vi "Script VeriStand Model core.vi"(9 "release/debug?":bool, 10 "build?":bool, 11 "VI path":path) -> (0 "error out":errorcluster)   [LabVIEW 2015, in "CD model script.lvlib"]
uses:
  CD model script.lvlib
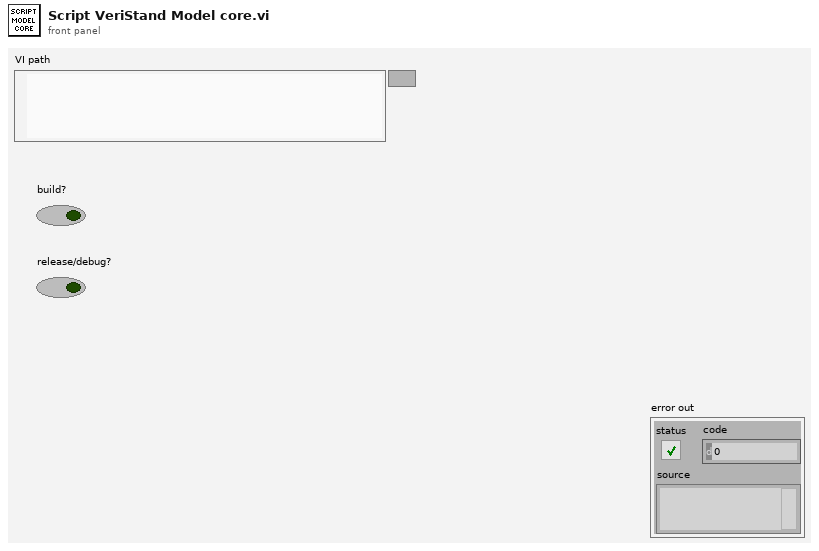
[diagram p1: front panel]
types:
  T1 = typedef "CD model script.lvlib/interface spec.ctl" = cluster{"name":string, "control reference":refnum<vi>}
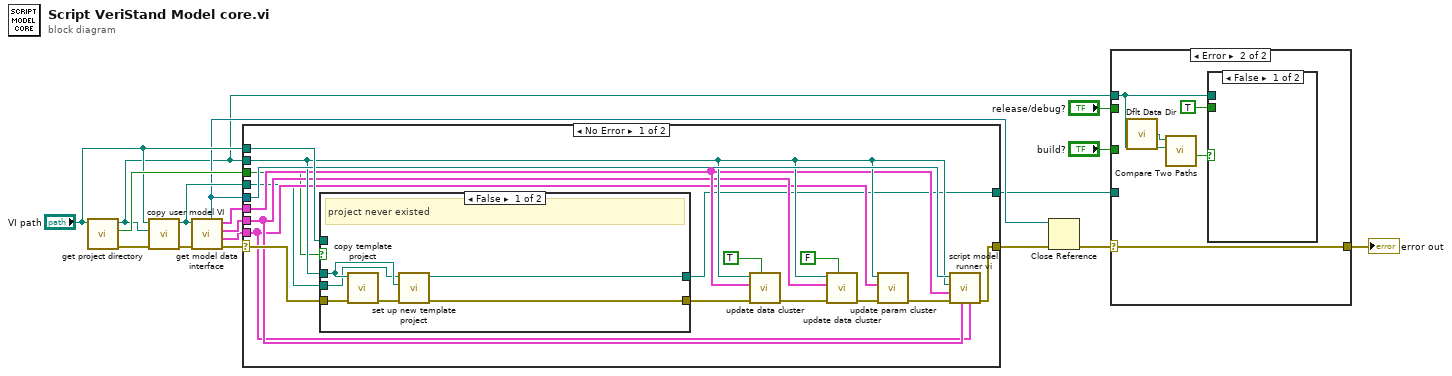
[diagram p0: block diagram]
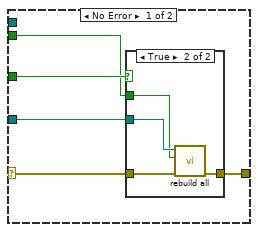
[diagram p2: hidden frame]
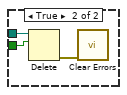
[diagram p4: hidden frame]
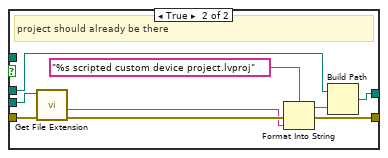
[diagram p5: hidden frame]
diagram:
  n1 = call "get project directory.vi"("VI path"="VI path") -> ("error out"=w15:errorcluster, "already existed"=w16:bool, "project directory"=w1:path)  [unwired: 8 in]
  n2 = call "copy user model VI.vi"("error in"=w15, "project directory"=w1, "VI path"="VI path") -> ("error out"=w12:errorcluster, "new VI path"=w11:path)  [unwired: 7 in]
  n3 = call "get model data interface.vi"("error in"=w12, "new VI path"=w11) -> ("error out"=w13:errorcluster, "parameters"=w8:T1[], "indicators"=w9:T1[], "controls"=w10:T1[], "vi reference"=w7:refnum<vi>)  [unwired: 5 in]
  n4 = case shown="No Error" w13 {
    selector: w13 -> [w34 w50]
    tunnel: w1 -> [w25 _]
    tunnel: [w19 w50] -> w17
    tunnel: w16 -> [w21 _]
    tunnel: "VI path" -> [w33 _]
    tunnel: w11 -> [w20 _]
    tunnel: w10 -> [w24 _]
    tunnel: w9 -> [w23 _]
    tunnel: w8 -> [w22 _]
    tunnel: w7 -> [w26 _]
    tunnel: [w18 _] -> w3
    frame No Error {
      n5 = case shown="False" w21 {
        tunnel: w25 -> [w37 w42]
        tunnel: [w39 w49] -> w32
        tunnel: w34 -> [w40 w48]
        tunnel: w33 -> [_ _]
        tunnel: w20 -> [w36 w44]
        tunnel: [w35 w41] -> w18
        frame False {
          # "project never existed"
          n6 = call "copy template project.vi"("error in"=w40, "project directory"=w37) -> ("error out"=w38:errorcluster)  [unwired: 9 in]
          n7 = call "set up new template project.vi"("error in"=w38, "project directory"=w37, "VI path"=w36) -> ("error out"=w39:errorcluster, "new project"=w35:path)  [unwired: 7 in]
        }
        frame True {
          # "project should already be there"
          n8 = call <vilib>:"Get File Extension.vi"("error in (no error)"=w48, "file"=w44) -> ("error out"=w45:errorcluster, "filename without extension"=w43:string)  [unwired: 5 in, 3 out]
          n9 = Format Into String(format string="%s scripted custom device project.lvproj", error in=w45, w43) -> (resulting string=w47:string, error out=w49:errorcluster)  [unwired: 1 in]
          n10 = Build Path(base path=w42, name or relative path=w47) -> (appended path=w41:path)
        }
      }
      n11 = call "update data cluster.vi"("inputs?"=TRUE, "error in"=w32, "controls"=w24, "project directory"=w25) -> ("error out"=w31:errorcluster)  [unwired: 7 in]
      n12 = call "update data cluster.vi"("inputs?"=FALSE, "error in"=w31, "controls"=w23, "project directory"=w25) -> ("error out"=w30:errorcluster)  [unwired: 7 in]
      n13 = call "update param cluster.vi"("error in (no error)"=w30, "controls"=w22, "project directory"=w25) -> ("error out"=w27:errorcluster)  [unwired: 8 in]
      n14 = call "script model runner vi.vi"("parameters"=w22, "indicators"=w23, "error in"=w27, "controls"=w24, "project directory"=w25, "VI in"=w26) -> ("error out"=w19:errorcluster)  [unwired: 5 in]
    }
    frame Error {
    }
  }
  n15 = Close Reference(reference=w7, error in (no error)=w17) -> (error out=w5:errorcluster)
  n16 = case shown="Error" w5 {
    selector: w5 -> [w54 w65]
    tunnel: [w55 w65] -> w6
    tunnel: "build?" -> [w53 _]
    tunnel: w3 -> [w52 _]
    tunnel: "release/debug?" -> [w51 _]
    tunnel: w1 -> [_ w63]
    frame No Error {
      n17 = case shown="True" w53 {
        tunnel: [w56 w59] -> w55
        tunnel: w54 -> [w56 w60]
        tunnel: w52 -> [_ w58]
        tunnel: w51 -> [_ w57]
        frame False {
        }
        frame True {
          n18 = call "rebuild all.vi"("error in (no error)"=w60, "release (T) /debug (F)"=w57, "project path"=w58) -> ("error"=w59:errorcluster)  [unwired: 8 in]
        }
      }
    }
    frame Error {
      n19 = call <vilib>:"Dflt Data Dir.vi"() -> ("App:Default Data Directory"=w62:path)
      n20 = call <vilib>:"Compare Two Paths.vi"("Path 2"=w63, "Path 1"=w62) -> ("Path 2 Relative to Path 1?"=w61:bool)  [unwired: 6 in, 3 out]
      n21 = case shown="False" w61 {
        tunnel: TRUE ("entire hierarchy (F)") -> [_ w67]
        tunnel: w63 -> [_ w66]
        frame False {
        }
        frame True {
          n22 = Delete(path (use dialog)=w66, entire hierarchy (F)=w67) -> (error out=w68:errorcluster)  [unwired: 3 in, 2 out]
          n23 = call <vilib>:"Clear Errors.vi"("error in (no error)"=w68) -> ()  [unwired: 5 in, 2 out]
        }
      }
    }
  }
  "error out" <- w6
